vi "Convert Channel Values to WSS Generate Digital Settings.vi"(9 "Length":i32, 10 "Index":i32, 11 "Channel Values in":dbl[](array[numeric])) -> (2 "WSS Generate Digital Settings":T1, 3 "Channel Values out":dbl[](array[numeric]))   [LabVIEW 2018, in "FPGA Addon Engine.lvlib"]
uses:
  FPGA Addon Engine.lvlib
  Submodules/Source/Types/WSS.Generate.Digital.Settings.ctl
  Submodules/Source/Speciality FPGA IO.lvlib
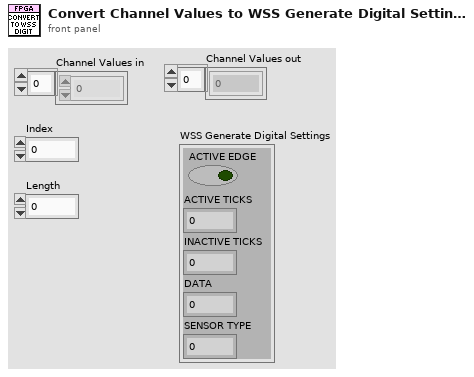
[diagram p1: front panel]
types:
  T1 = typedef "Speciality FPGA IO.lvlib/WSS.Generate.Digital.Settings.ctl" = cluster{"ACTIVE EDGE":bool, "ACTIVE TICKS":u32, "INACTIVE TICKS":u32, "DATA":u8, "SENSOR TYPE":u8}
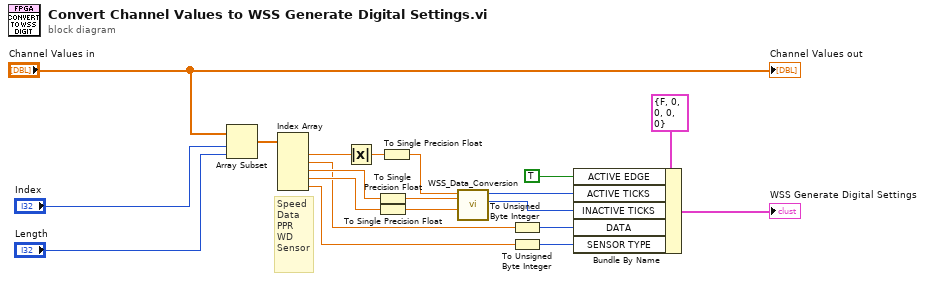
[diagram p0: block diagram]
diagram:
  # "Speed\nData\nPPR\nWD\nSensor"
  n1 = Array Subset(array="Channel Values in", index="Index", length="Length") -> (w1:dbl[])
  n2 = Index Array(array=w1) -> (element #1=w3:dbl, element #2=w4:dbl, element #3=w5:dbl, element #4=w6:dbl, element #5=w7:dbl)  [unwired: 5 in]
  n3 = Absolute Value(x=w3) -> (abs(x)=w15:dbl)
  n4 = To Single Precision Float(number=w5) -> (single precision float=w11:sgl)
  n5 = To Single Precision Float(number=w6) -> (single precision float=w12:sgl)
  n6 = To Single Precision Float(number=w15) -> (single precision float=w10:sgl)
  n7 = call "WSS_Data_Conversion.vi"("WD"=w12, "PPR"=w11, "Speed"=w10) -> ("Inactive"=w14:u32, "Active"=w13:u32)  [unwired: 7 in]
  n8 = To Unsigned Byte Integer(number=w4) -> (unsigned 8bit integer=w9:u8)
  n9 = To Unsigned Byte Integer(number=w7) -> (unsigned 8bit integer=w8:u8)
  n10 = Bundle By Name(cluster=T1 {"ACTIVE EDGE"=FALSE, "ACTIVE TICKS"=0, "INACTIVE TICKS"=0, "DATA"=0, "SENSOR TYPE"=0} ("Settings"), "ACTIVE EDGE"=TRUE, "ACTIVE TICKS"=w13, "INACTIVE TICKS"=w14, "DATA"=w9, "SENSOR TYPE"=w8) -> (→"WSS Generate Digital Settings":T1)
  "Channel Values out" <- "Channel Values in"
